vi "Exercise 4 Solution.vi"() -> ()   [LabVIEW 2019]
panel:
  in  "B":i32=5
  in  "A":i32=3
  out "Output Array":string[][](array[string])
  # "X: n mod(A) == 0 OR n mod(B) == 0\nO: n mod(A) == 0 AND n mod(B) == 0"
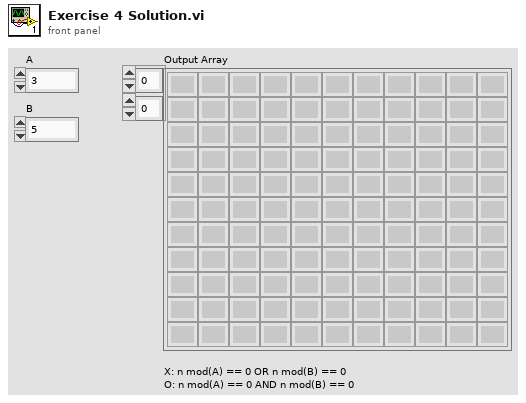
[diagram p1: front panel]
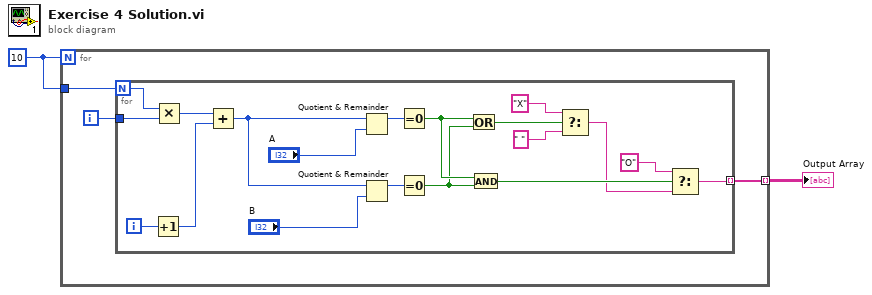
[diagram p0: block diagram]
diagram:
  w1 = 10
  n1 = for {
    N: w1 -> [_]
    tunnel: [w5] -> w2 mode=indexing
    tunnel: w1 -> [w3]
    i -> [w4]
    n2 = for {
      N: w3 -> [w10]
      tunnel: [w12] -> w5 mode=indexing
      tunnel: w4 -> [w11]
      i -> [w9]
      n3 = Increment(x=w9) -> (x+1=w7:i32)
      n4 = Multiply(x=w10, y=w11) -> (x*y=w8:i32)
      n5 = Add(x=w8, y=w7) -> (x+y=w6:i32)
      n6 = Quotient & Remainder(x=w6, y="A") -> (x-y*floor(x/y)=w22:i32)  [unwired: 1 out]
      n7 = Quotient & Remainder(x=w6, y="B") -> (x-y*floor(x/y)=w21:i32)  [unwired: 1 out]
      n8 = Equal To 0?(x=w22) -> (x = 0?=w20:bool)
      n9 = Equal To 0?(x=w21) -> (x = 0?=w19:bool)
      n10 = Or(x=w20, y=w19) -> (x .or. y?=w18:bool)
      n11 = And(x=w20, y=w19) -> (x .and. y?=w15:bool)
      n12 = Select(t="X", s=w18, f=" ") -> (s? t:f=w13:string)
      n13 = Select(t="O", s=w15, f=w13) -> (s? t:f=w12:string)
    }
  }
  "Output Array" <- w2
